vi "ConfigMeasurement.vi"(8 "error in (no error)":errorcluster, 11 "NiPxi6123 in":refnum<class "NiPxi6123.lvclass">) -> (0 "error out":errorcluster, 3 "NiPxi6123 out":refnum<class "NiPxi6123.lvclass">)   [LabVIEW 2014, in "SamplerPlugins.lvlib" / "NiPxi6123.lvclass"]
uses:
  NiPxi6123.lvclass
  <vilib>/DAQmx/create/channels.llb/DAQmx Create Channel (AI-Voltage-Basic).vi
  <vilib>/DAQmx/create/channels.llb/DAQmx Create Channel (AI-Voltage-RMS).vi
  <vilib>/ErrorRing/Error Ring.xnode
  <vilib>/Utility/error.llb/Error Cluster From Error Code.vi
  <vilib>/DAQmx/create/channels.llb/DAQmx Create Channel (AI-Current-Basic).vi
  <vilib>/DAQmx/create/channels.llb/DAQmx Create Channel (AI-Current-RMS).vi
  <vilib>/DAQmx/create/channels.llb/DAQmx Create Channel (AI-Frequency-Voltage).vi
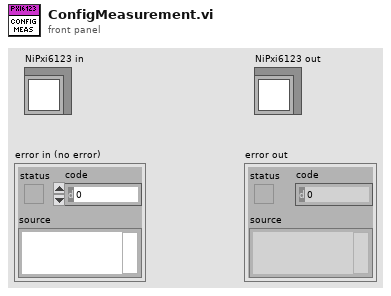
[diagram p1: front panel]
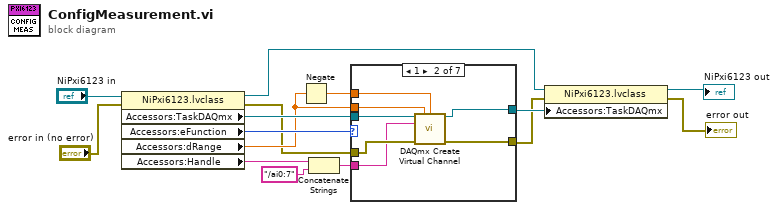
[diagram p0: block diagram]
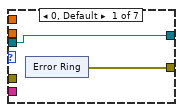
[diagram p2: hidden frame]
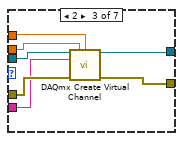
[diagram p3: hidden frame]
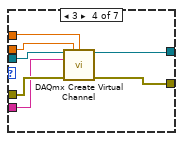
[diagram p4: hidden frame]
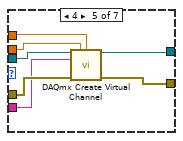
[diagram p5: hidden frame]
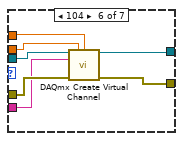
[diagram p6: hidden frame]
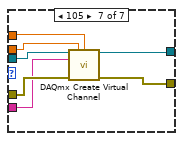
[diagram p7: hidden frame]
diagram:
  n1 = property class="NiPxi6123.lvclass"(reference="NiPxi6123 in", error in="error in (no error)") -> (reference out=w7:refnum<class "NiPxi6123.lvclass">, error out=w9:errorcluster, "Accessors:TaskDAQmx"=w12:refnum<k21>, "Accessors:eFunction"=w13:u16, "Accessors:dRange"=w11:dbl, "Accessors:Handle"=w3:string)
  n2 = Negate(x=w11) -> (-x=w10:dbl)
  n3 = Concatenate Strings(w3, "/ai0:7" ("regular expression")) -> (w1:string)
  n4 = case shown="1" w13 {
    tunnel: w12 -> [w16 w29 w34 w41 w48 w55 w62]
    tunnel: w11 -> [_ w28 w35 w42 w49 w56 w63]
    tunnel: w10 -> [_ w27 w36 w43 w50 w57 w64]
    tunnel: w9 -> [_ w26 w33 w40 w47 w54 w61]
    tunnel: [w17 w25 w32 w39 w46 w53 w60] -> w5
    tunnel: [w16 w24 w31 w38 w45 w52 w59] -> w6
    tunnel: w1 -> [_ w23 w30 w37 w44 w51 w58]
    frame 0, Default {
      n5 = xnode "Error Ring"() -> ("error out"=w17:errorcluster)
    }
    frame 1 {
      n6 = call-poly <vilib>:"DAQmx Create Virtual Channel.vi"("task in"=w29, "maximum value"=w28, "minimum value"=w27, "physical channels"=w23, "error in"=w26) -> ("task out"=w24:refnum<k21>, "error out"=w25:errorcluster)  [unwired: 9 in]
    }
    frame 2 {
      n7 = call-poly <vilib>:"DAQmx Create Virtual Channel.vi"("task in"=w34, "maximum value"=w35, "minimum value"=w36, "physical channels"=w30, "error in"=w33) -> ("task out"=w31:refnum<k21>, "error out"=w32:errorcluster)  [unwired: 9 in]
    }
    frame 3 {
      n8 = call-poly <vilib>:"DAQmx Create Virtual Channel.vi"("task in"=w41, "maximum value"=w42, "minimum value"=w43, "physical channels"=w37, "error in"=w40) -> ("task out"=w38:refnum<k21>, "error out"=w39:errorcluster)  [unwired: 9 in]
    }
    frame 4 {
      n9 = call-poly <vilib>:"DAQmx Create Virtual Channel.vi"("task in"=w48, "maximum value"=w49, "minimum value"=w50, "physical channels"=w44, "error in"=w47) -> ("task out"=w45:refnum<k21>, "error out"=w46:errorcluster)  [unwired: 9 in]
    }
    frame 104 {
      n10 = call-poly <vilib>:"DAQmx Create Virtual Channel.vi"("task in"=w55, "maximum value"=w56, "minimum value"=w57, "physical channels"=w51, "error in"=w54) -> ("task out"=w52:refnum<k21>, "error out"=w53:errorcluster)  [unwired: 9 in]
    }
    frame 105 {
      n11 = call-poly <vilib>:"DAQmx Create Virtual Channel.vi"("task in"=w62, "maximum value"=w63, "minimum value"=w64, "physical channels"=w58, "error in"=w61) -> ("task out"=w59:refnum<k21>, "error out"=w60:errorcluster)  [unwired: 9 in]
    }
  }
  n12 = property class="NiPxi6123.lvclass"(reference=w7, error in=w5, "Accessors:TaskDAQmx"=w6) -> (reference out=→"NiPxi6123 out":refnum<class "NiPxi6123.lvclass">, error out=→"error out":errorcluster)
